vi "CurveEditor.vi"(8 "error in (no error)":errorcluster caption="entrée d'erreur (pas d'erreur)", 9 "Experiment.lvclass":refnum<class "Experiment.lvclass">=refnum, 11 "Interface en entrée":refnum<class "Interface.lvclass"> caption="Interface Class in") -> (0 "error out":errorcluster caption="sortie d'erreur", 1 "Experiment.lvclass Out":refnum<class "Experiment.lvclass">, 3 "Interface en sortie":refnum<class "Interface.lvclass"> caption="Interface Class out")   [LabVIEW 2019, in "Interface.lvclass"]
uses:
  Interface.lvclass
  Experiment Class/Experiment.lvclass
  DevicesClass/Tools/Tools.lvclass
  Calculations Class/DefaultDev_Func.ctl
  CurveSetup.ctl
  CrvEdStates.ctl
  Interface.lvclass/Interface.ctl
  <vilib>/Utility/error.llb/DialogType.ctl
  Calculations Class/Calculations.lvclass
panel:
  out "Current Task":i32=-1
  out "ScanInd":i32
  in  "AddDataSrc":bool
  in  "EditSource":i32(listbox) caption="Editing Source Curves"
  in  "Data Source 2":i32(listbox) caption="Added Operations"
  out "PanelViRefOut":refnum<vi>[](array[refnum])
  out "Point Count":i32
  out "Curve Preview":cluster{dbl[], dbl[]}[](graph)
  in  "ScanDatSrc":bool[](array[boolean])
  in  "RemOper":bool
  in  "RemDataSrc":bool
  in  "EditTask":i32(listbox) caption="Editing Task"
  in  "AddAqData":bool
  in  "Acquired Data List":i32[](listbox)
  out "2D Scan":bool
  in  "2D Plot Act":bool caption="2D Plot"
  in  "Data Only":bool
  out "GraphIndex":i32
  in  "CreateOper":bool
  in  "SaveCurvePar":bool
  in  "DisplayName":string
  out "CrvParOut":T1[](array[typedef])
  out "NomDon":string[](array[string])=["RTêta;", "X&Y;"]
  out "VarParams":string[][](array[string])
  in  "ScanParam":u16(ring) caption="Scan Parameter"
  in  "Operation":T2
  in  "stop":bool
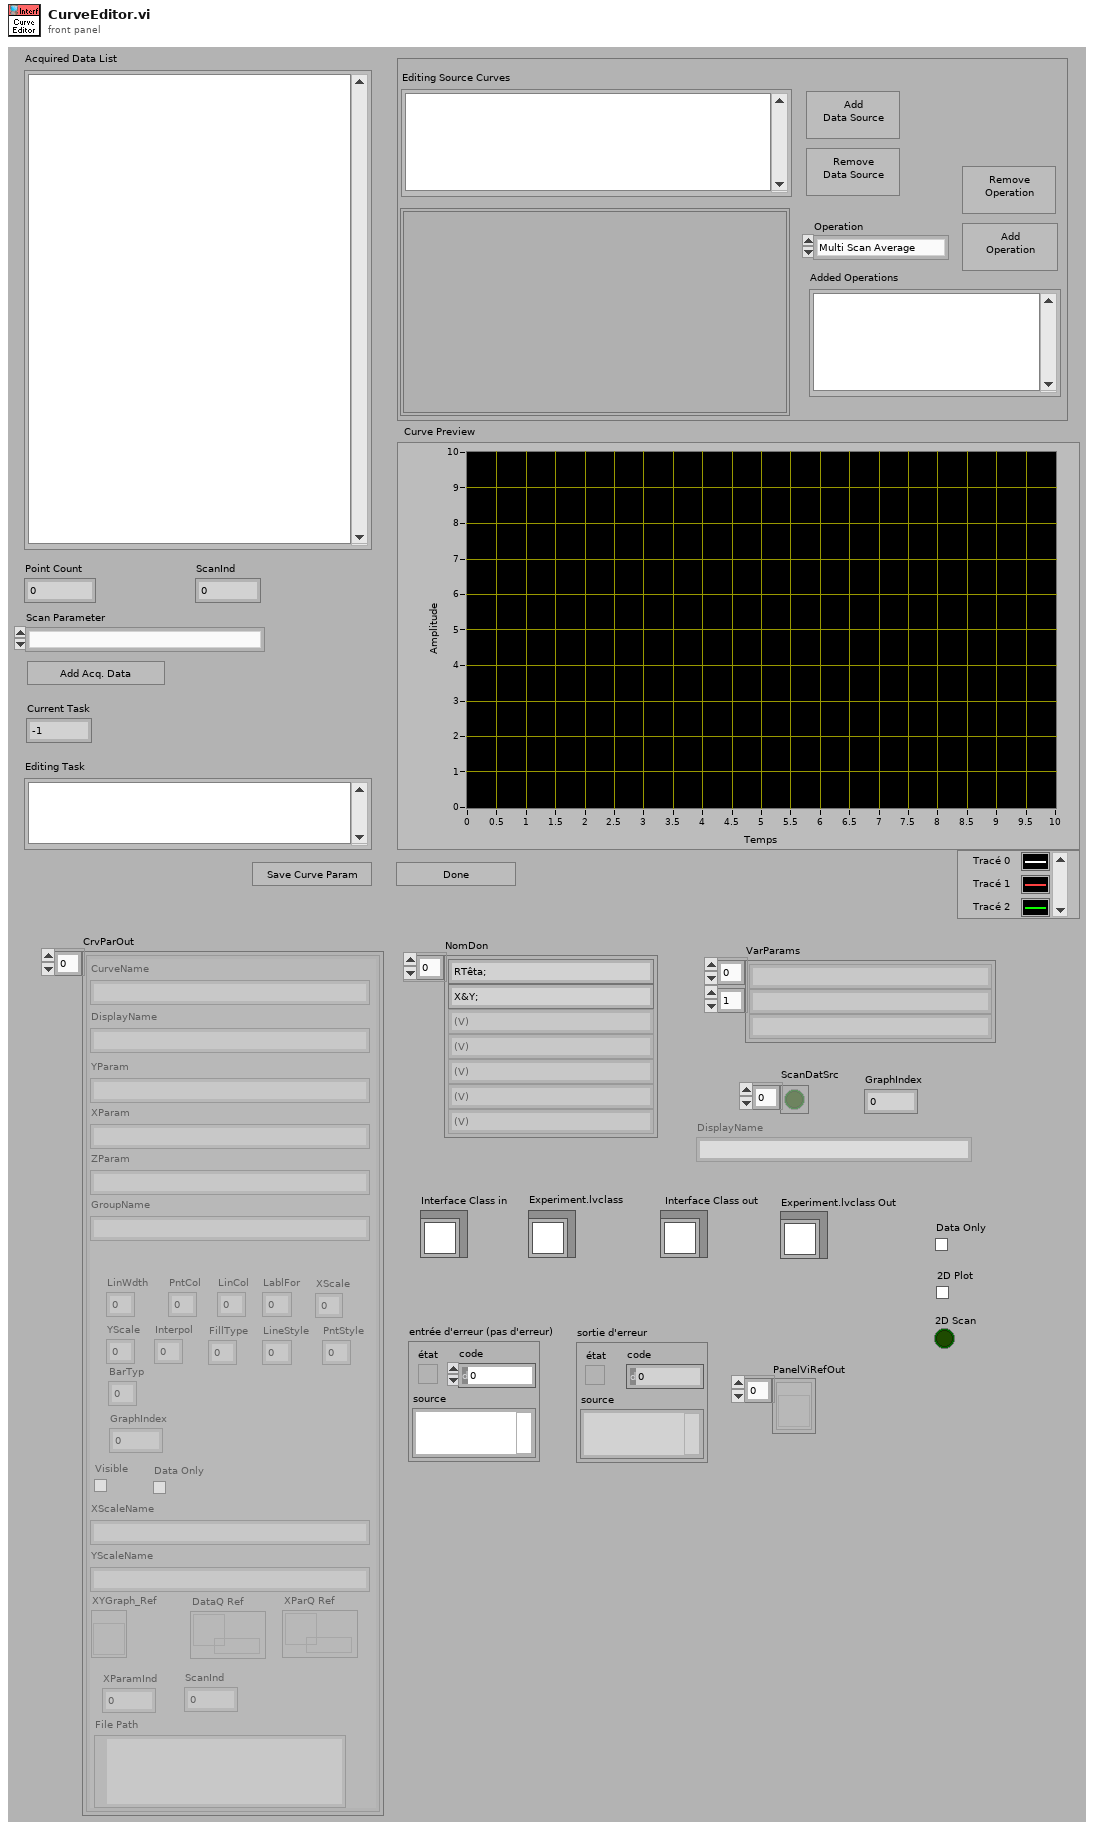
[diagram p1: front panel]
types:
  T1 = typedef "Interface.lvclass/CurveSetup.ctl" = cluster{"CurveName":string, "YParam":string, "XParam":string, "ZParam ":string, "GroupName":string, "LinWdth":u8, "PntCol":u32, "LinCol":u32, "LablFor":u8, "XScale":u32, "YScale":u32, "Interpol":u8, "DisplayName":string, "FillType":i16, "LineStyle":u8, "PntStyle":u8, "BarTyp":u8, "GraphIndex":i32, "Visible":bool, "XScaleName":string, "YScaleName":string, "XYGraph_Ref":refnum<vi>, "Data Only":bool, "DataQ Ref":refnum<queue>, "XParQ Ref":refnum<queue>, "XParamInd":i32, "ScanInd":i32, "File Path":path}
  T2 = typedef "Calculations.lvclass/DefaultDev_Func.ctl" = enum16{"Multi Scan Average", "Running Average", "Summ"}
  T3 = typedef "CrvEdStates.ctl" = enum16{"InitProg", "CreateCalc", "SaveParams", "Error", "Stop"}
  T4 = typedef "DialogType.ctl" = u16
  T5 = typedef "Interface.lvclass/ScanParams.ctl" = cluster{"Entête":string, "Scan list":string[], "NbCourbe":i32, "IndCourbe":i64, "NomDon":string[], "Session ":i32, "Date":string, "Time":string, "VarParams":string[][], "UserName":string, "ScanTableSize":i32[], "VarPar list":string[], "DescKeyword":string}
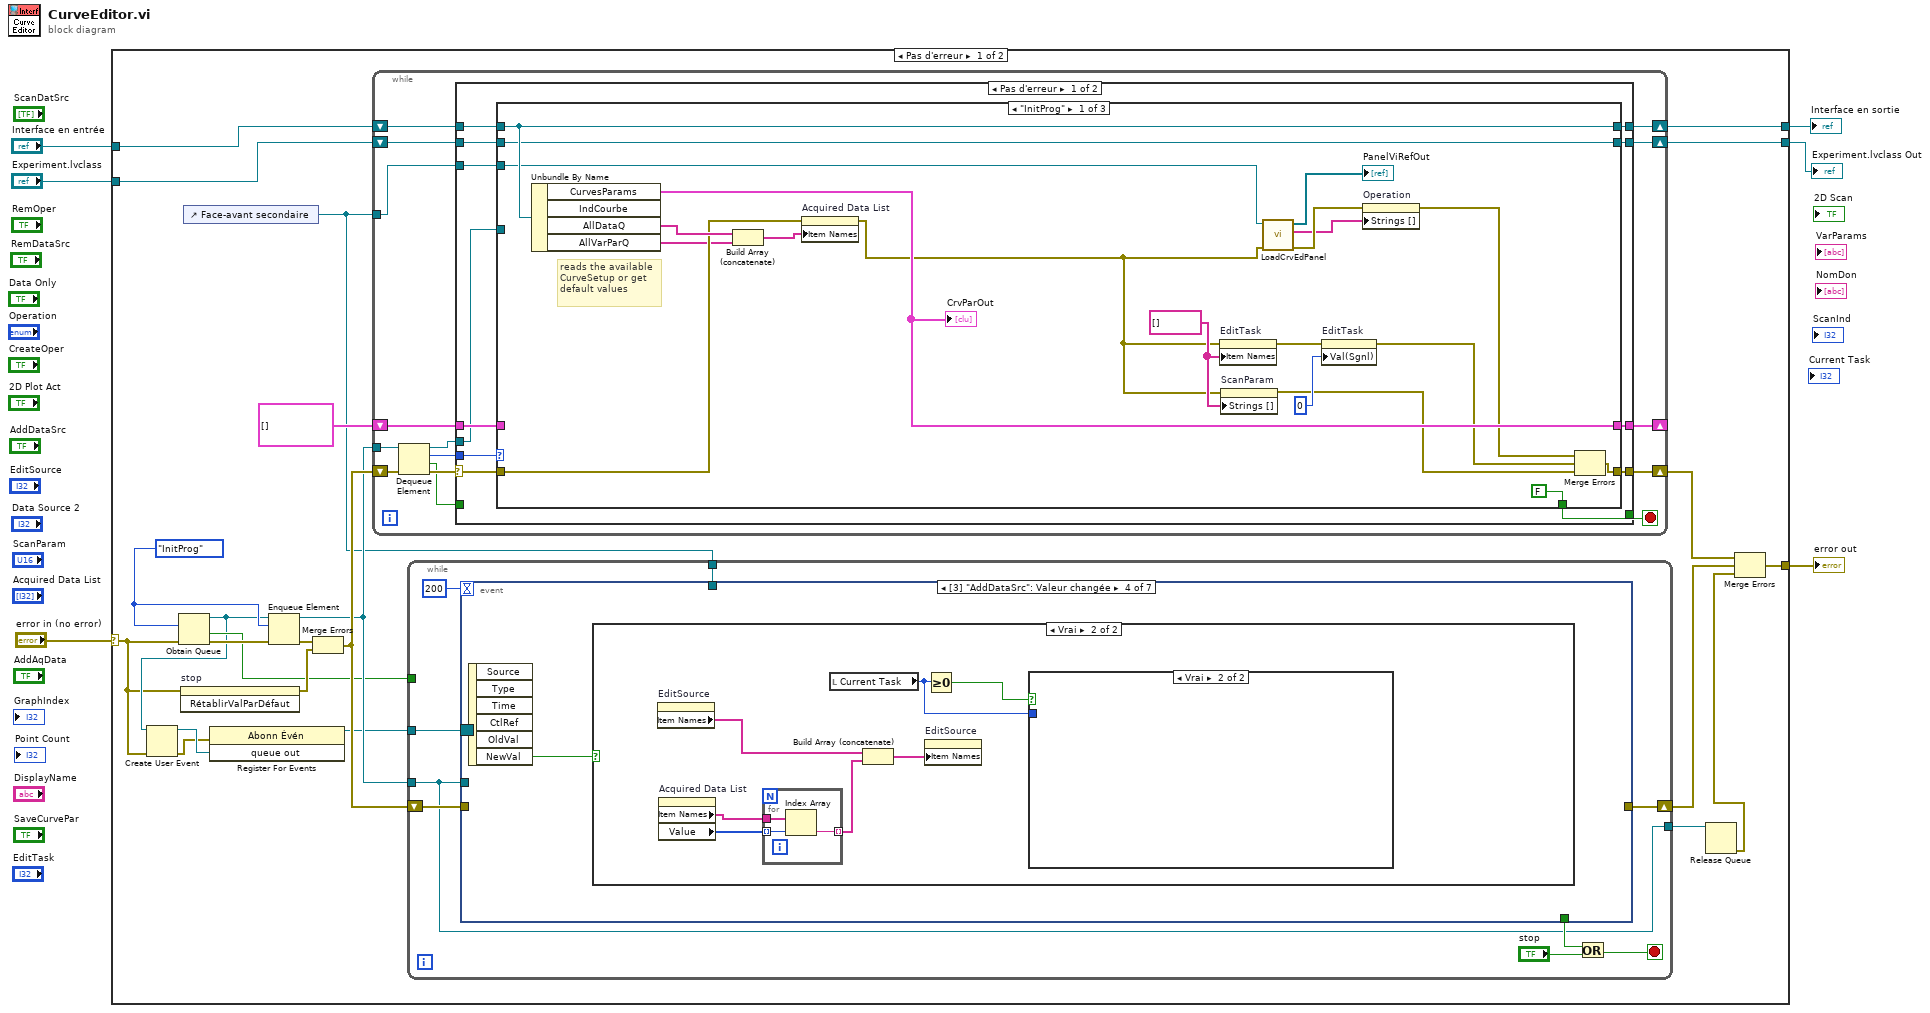
[diagram p0: block diagram]
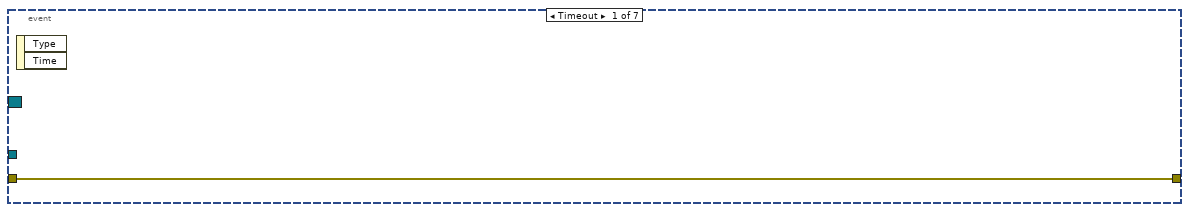
[diagram p2: hidden frame]
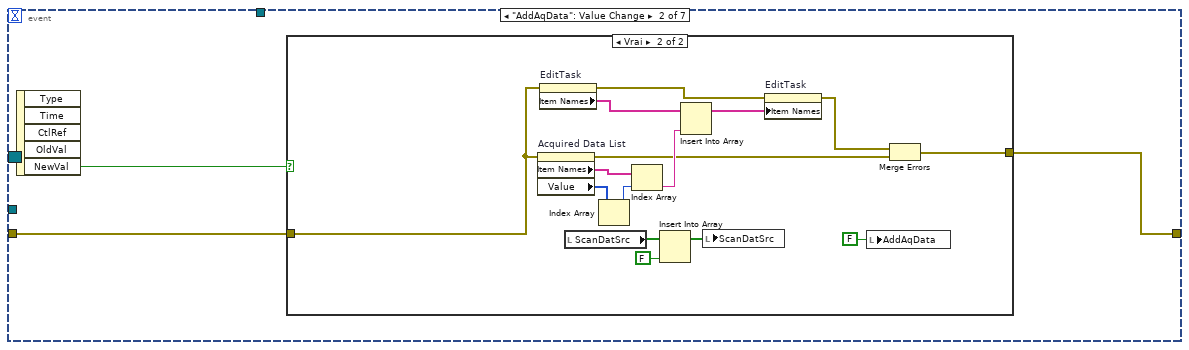
[diagram p3: hidden frame]
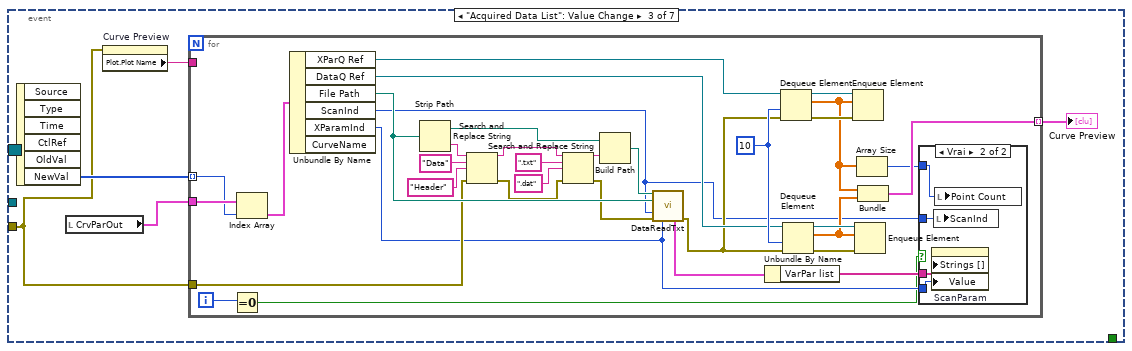
[diagram p5: hidden frame]
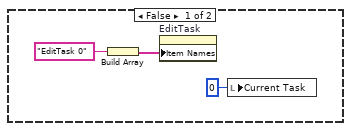
[diagram p8: hidden frame]
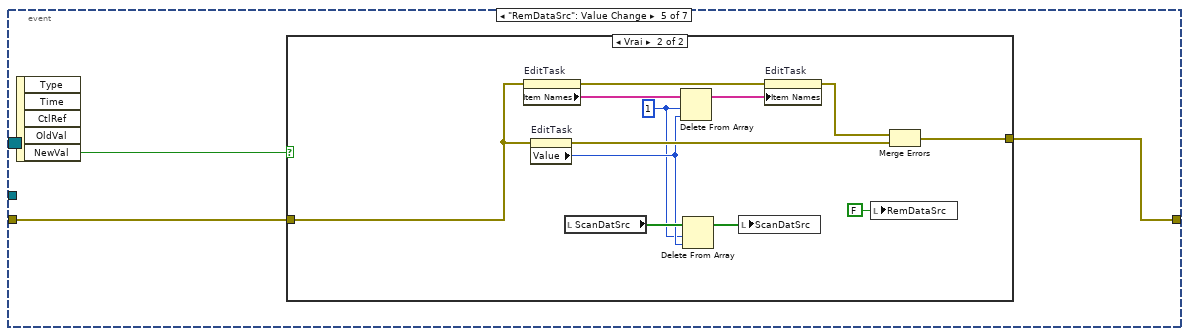
[diagram p9: hidden frame]
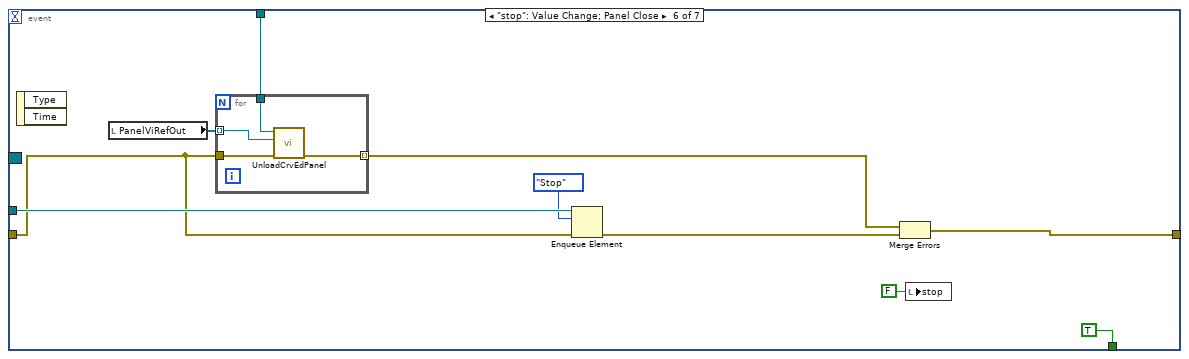
[diagram p11: hidden frame]
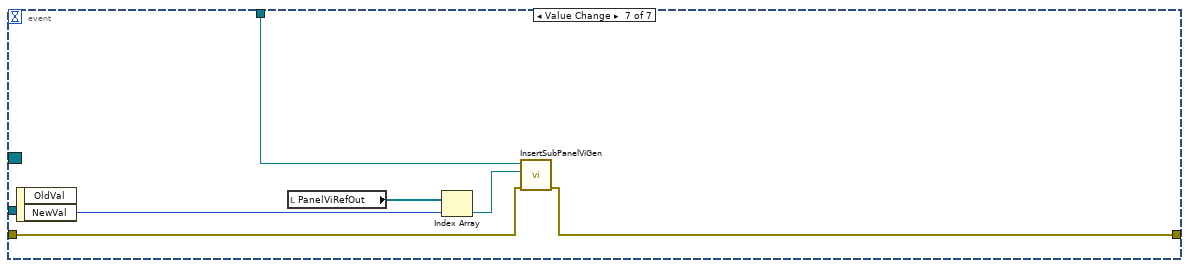
[diagram p12: hidden frame]
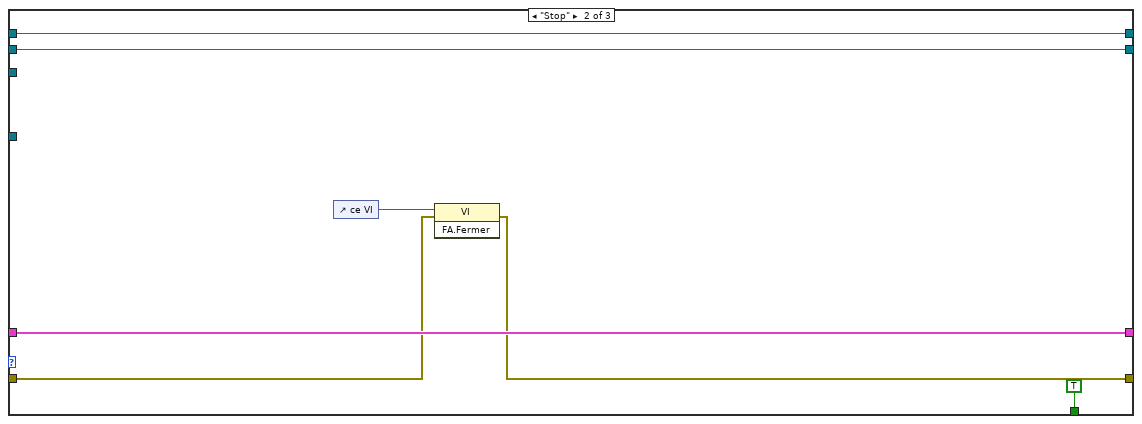
[diagram p13: hidden frame]
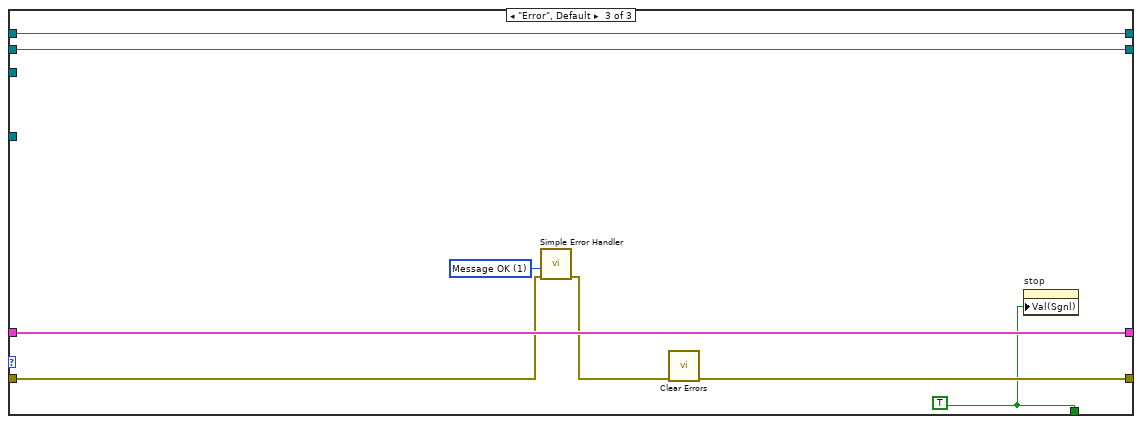
[diagram p14: hidden frame]
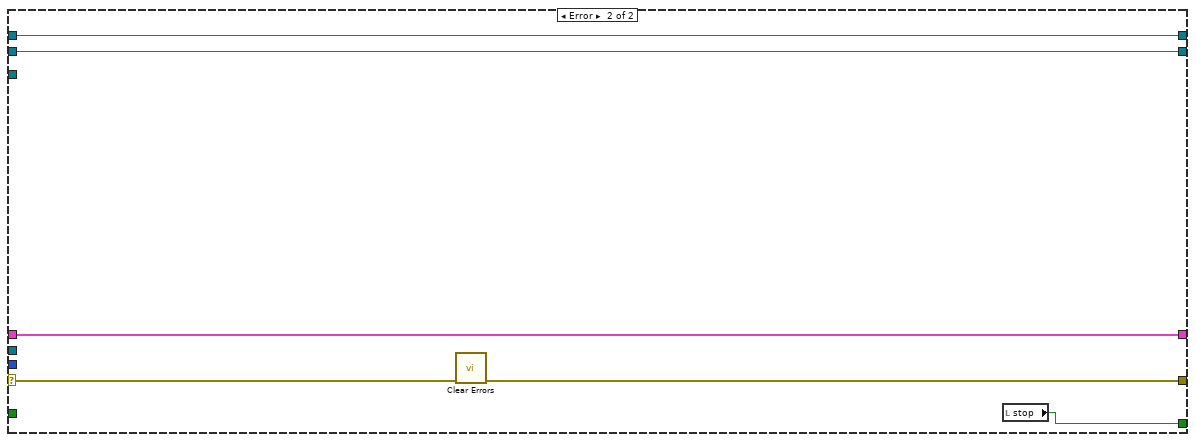
[diagram p15: hidden frame]
diagram:
  n1 = case shown="Pas d'erreur" "error in (no error)" {
    selector: "error in (no error)" -> [w11 w222]
    tunnel: [w20 w222] -> w5
    tunnel: "Interface en entrée" -> [w23 w221]
    tunnel: [w18 w221] -> w3
    tunnel: "Experiment.lvclass" -> [w28 w220]
    tunnel: [w19 w220] -> w1
    frame No Error {
      w14 = CrvEdStates."InitProg" ("Énum")
      n2 = Obtain Queue(element data type=w14, error in (no error)=w11) -> (queue out=w12:refnum<queue>, created new?=w15:bool, error out=w29:errorcluster)  [unwired: 3 in]
      n3 = Create User Event(user event datatype=w12, error in=w11) -> (user event=w10:refnum<user-event>, error out=w9:errorcluster)
      n4 = invoke on="stop" class="Bool (strict)" method="RétablirValParDéfaut"(error in=w11) -> (error out=w25:errorcluster)  [unwired: 2 in, 2 out]
      n5 = control-ref of="Face-avant secondaire"() -> (w7:refnum<vi>)
      n6 = register-events(error in=w9, w10) -> (reference out=w8:refnum<event-registration>)  [unwired: 1 in, 1 out]
      n7 = Enqueue Element(queue=w12, element=w14, error in (no error)=w29) -> (queue out=w17:refnum<queue>, error out=w26:errorcluster)  [unwired: 1 in, 1 out]
      n8 = Merge Errors(w26, w25) -> (w24:errorcluster)
      n9 = while {
        shift-right: [w160] -> w21
        shift-left: w24 -> [w166]
        tunnel: w17 -> [w157]
        shift-right: [w161] -> w18
        shift-left: w23 -> [w164]
        shift-right: [w163] -> w19
        shift-left: w28 -> [w165]
        shift-right: [w159] -> _
        shift-left: T1[] [] ("CurveParamsOut") -> [w158]
        tunnel: w7 -> [w156]
        stop <- w162 stop-if-true
        n10 = Dequeue Element(queue=w157, error in (no error)=w166) -> (queue out=w153:refnum<queue>, element=w155:T3, timed out?=w152:bool, error out=w154:errorcluster)  [unwired: 1 in]
        n11 = case shown="Pas d'erreur" w154 {
          selector: w154 -> [w168 w219]
          tunnel: w165 -> [w178 w216]
          tunnel: w164 -> [w177 w217]
          tunnel: [w176 w216] -> w163
          tunnel: [w175 w214] -> w162
          tunnel: [w174 w217] -> w161
          tunnel: [w173 w215] -> w160
          tunnel: [w172 w218] -> w159
          tunnel: w158 -> [w171 w218]
          tunnel: w156 -> [w170 _]
          tunnel: w155 -> [w169 _]
          tunnel: w153 -> [w167 _]
          tunnel: w152 -> [_ _]
          frame No Error {
            n12 = case shown="\"InitProg\"" w169 {
              tunnel: w178 -> [w191 w204 w211]
              tunnel: w177 -> [w197 w203 w212]
              tunnel: w168 -> [w189 w200 w210]
              tunnel: [w191 w204 w211] -> w176
              tunnel: [FALSE TRUE w206] -> w175
              tunnel: [w197 w203 w212] -> w174
              tunnel: [w196 w199 w208] -> w173
              tunnel: [w192 w202 w213] -> w172
              tunnel: w171 -> [_ w202 w213]
              tunnel: w167 -> [_ _ _]
              tunnel: w170 -> [w183 _ _]
              frame "InitProg" {
                w187 = string[] [] ("Item Names")
                # "reads the available CurveSetup or get default values"
                n13 = Unbundle By Name(w197) -> ("CurvesParams"=w192:T1[], "AllDataQ"=w193:string[], "AllVarParQ"=w185:string[])  [unwired: 1 out]
                "CrvParOut" <- w192
                n14 = Build Array (concatenate)(w193, w185) -> (w186:string[])
                n15 = property on="Acquired Data List" class="LstDér (strict)"(error in=w189, "Item Names"=w186) -> (error out=w184:errorcluster)  [unwired: 1 in, 1 out]
                n16 = property on="EditTask" class="LstDér (strict)"(error in=w184, "Item Names"=w187) -> (error out=w195:errorcluster)  [unwired: 1 in, 1 out]
                n17 = property on="ScanParam" class="MDér (strict)"(error in=w184, "Strings []"=w187) -> (error out=w188:errorcluster)  [unwired: 1 in, 1 out]
                n18 = call "LoadCrvEdPanel.vi"("error in (no error)"=w184, "RemPanRef"=w183) -> ("sortie d'erreur"=w182:errorcluster, "ViNameOut"=w181:string[], "PanelViRefOut"=→"PanelViRefOut":refnum<vi>[])  [unwired: 7 in]
                n19 = property on="EditTask" class="LstDér (strict)"(error in=w195, "Val(Sgnl)"=0 ("Valeur (Signalisation)")) -> (error out=w190:errorcluster)  [unwired: 1 in, 1 out]
                n20 = property on="Operation" class="Énum (strict)"(error in=w182, "Strings []"=w181) -> (error out=w180:errorcluster)  [unwired: 1 in, 1 out]
                n21 = Merge Errors(w180, w190, w188) -> (w196:errorcluster)
              }
              frame "Stop" {
                n22 = control-ref of="ce VI"() -> (w201:refnum<vi>)
                n23 = invoke class="VI" method="FA.Fermer"(reference=w201, error in=w200) -> (error out=w199:errorcluster)  [unwired: 1 in, 2 out]
              }
              frame "Error", Default {
                w206 = TRUE
                w207 = T4 1 items=["pas de dialogue", "Message OK", "Message continuer ou arrêter", "Message OK + mises en garde", "Arrêter/Continuer + mises en garde"] ("type of dialog (OK msg:1)")
                n24 = call <vilib>:"Simple Error Handler.vi"("type of dialog (OK msg:1)"=w207, "error in (no error)"=w210) -> ("error out"=w209:errorcluster)  [unwired: 3 in, 4 out]
                n25 = call <vilib>:"Clear Errors.vi"("error in (no error)"=w209) -> ("error out"=w208:errorcluster)  [unwired: 5 in, 1 out]
                n26 = property on="stop" class="Bool (strict)"("Val(Sgnl)"=w206) -> ()  [unwired: 2 in, 2 out]
              }
            }
          }
          frame Error {
            n27 = call <vilib>:"Clear Errors.vi"("error in (no error)"=w219) -> ("error out"=w215:errorcluster)  [unwired: 5 in, 1 out]
            n28 = local read "stop"() -> (w214:bool)
          }
        }
      }
      n29 = while {
        shift-right: [w36] -> w22
        shift-left: w24 -> [w37]
        tunnel: w17 -> [w32]
        tunnel: w15 -> [_]
        tunnel: [w32] -> w13
        tunnel: w8 -> [w31]
        tunnel: w7 -> [w30]
        stop <- w34 stop-if-true
        n30 = event shown="[3] \"AddDataSrc\": Valeur changée" {
          selector: w31 -> [_ _ _ _ _ _ _]
          dyn-events: _ -> [_ _ _ _ _ _ _]
          timeout: 200 -> [_ _ _ _ _ _ _]
          tunnel: w32 -> [_ _ _ _ _ w140 _]
          tunnel: w37 -> [w39 w41 w60 _ w117 w135 w150]
          tunnel: [w39 w40 _ _ w116 w136 w149] -> w36
          tunnel: [_ _ _ _ _ TRUE _] -> w33
          tunnel: w30 -> [_ _ _ _ _ w132 w151]
          event Timeout {
            n31 = event-data() -> ()  [unwired: 1 in, 2 out]
          }
          event "AddAqData": Value Change {
            n32 = event-data() -> ("NewVal"=w42:bool)  [unwired: 1 in, 4 out]
            n33 = case shown="Vrai" w42 {
              tunnel: w41 -> [w43 w51]
              tunnel: [w43 w50] -> w40
              frame False {
              }
              frame True {
                n34 = property on="Acquired Data List" class="LstDér (strict)"(error in=w51) -> (error out=w52:errorcluster, "Item Names"=w58:string[], "Value"=w45:i32[])  [unwired: 1 in, 1 out]
                n35 = property on="EditTask" class="LstDér (strict)"(error in=w51) -> (error out=w54:errorcluster, "Item Names"=w56:string[])  [unwired: 1 in, 1 out]
                n36 = local read "ScanDatSrc"() -> (w48:bool[])
                n37 = Index Array(array=w45) -> (element=w44:i32)  [unwired: 1 in]
                n38 = Index Array(array=w58, index=w44) -> (element=w57:string)
                n39 = Insert Into Array(array=w48, new element=FALSE ("new element/subarray")) -> (w47:bool[])  [unwired: 1 in]
                n40 = Insert Into Array(array=w56, new element=w57) -> (w55:string[])  [unwired: 1 in]
                n41 = local write "ScanDatSrc"(w47) -> ()
                n42 = property on="EditTask" class="LstDér (strict)"(error in=w54, "Item Names"=w55) -> (error out=w53:errorcluster)  [unwired: 1 in, 1 out]
                n43 = local write "AddAqData"(FALSE ("AddAqData")) -> ()
                n44 = Merge Errors(w53, w52) -> (w50:errorcluster)
              }
            }
          }
          event "Acquired Data List": Value Change {
            n45 = event-data() -> ("NewVal"=w61:i32[])  [unwired: 1 in, 5 out]
            n46 = local read "CrvParOut"() -> (w63:T1[])
            n47 = property on="Curve Preview" class="GraphXY (strict)"(error in=w60) -> ("Plot.Plot Name"=w59:string)  [unwired: 1 in, 2 out]
            n48 = for {
              tunnel: w63 -> [w97]
              tunnel: [w87] -> w62 mode=indexing
              tunnel: w60 -> [w78]
              tunnel: w61 -> [w66] mode=indexing
              tunnel: w59 -> [_]
              i -> [w65]
              w92 = 10 ("timeout en ms (-1)")
              n49 = Equal To 0?(x=w65) -> (x = 0?=w64:bool)
              n50 = Index Array(array=w97, index=w66) -> (element=w96:T1)
              n51 = Unbundle By Name(w96) -> ("XParQ Ref"=w89:refnum<queue>, "DataQ Ref"=w88:refnum<queue>, "File Path"=w85:path, "ScanInd"=w67:i32, "XParamInd"=w70:i32)  [unwired: 1 out]
              n52 = Strip Path(path=w85) -> (stripped path=w81:path, name=w84:string)
              n53 = Search and Replace String(input string=w84, search string="Data" ("chaîne recherchée"), replace string="Header" ("chaîne de remplacement (\"\")"), error in=w78) -> (result string=w75:string, error out=w77:errorcluster)  [unwired: 4 in, 2 out]
              n54 = Search and Replace String(input string=w75, search string=".txt" ("chaîne recherchée"), replace string=".dat" ("chaîne de remplacement (\"\")"), error in=w77) -> (result string=w73:string, error out=w74:errorcluster)  [unwired: 4 in, 2 out]
              n55 = Build Path(base path=w81, name or relative path=w73) -> (appended path=w80:path)
              n56 = call "DataReadTxt.vi"("Chemin Header"=w80, "chemin Data"=w85, "ScanlistIndex"=w67, "error in"=w74, "VarParIndex"=w70) -> ("enregistrement(s)"=w72:T5, "error out"=w86:errorcluster)  [unwired: 3 in, 6 out]
              n57 = Unbundle By Name(w72) -> ("VarPar list"=w71:string[])
              n58 = Dequeue Element(queue=w89, timeout in ms (-1)=w92, error in (no error)=w86) -> (queue out=w95:refnum<queue>, element=w69:dbl[], error out=w91:errorcluster)  [unwired: 1 out]
              n59 = Dequeue Element(queue=w88, timeout in ms (-1)=w92, error in (no error)=w86) -> (queue out=w93:refnum<queue>, element=w90:dbl[], error out=w94:errorcluster)  [unwired: 1 out]
              n60 = Enqueue Element(queue=w95, element=w69, error in (no error)=w91) -> ()  [unwired: 1 in, 3 out]
              n61 = Enqueue Element(queue=w93, element=w90, error in (no error)=w94) -> ()  [unwired: 1 in, 3 out]
              n62 = Array Size(array=w69) -> (size(s)=w68:i32)
              n63 = Bundle(w69, w90) -> (w87:cluster{dbl[], dbl[]})  [unwired: 1 in]
              n64 = case shown="Vrai" w64 {
                tunnel: w71 -> [_ w101]
                tunnel: w70 -> [_ w100]
                tunnel: w68 -> [_ w99]
                tunnel: w67 -> [_ w98]
                frame False {
                }
                frame True {
                  n65 = property on="ScanParam" class="MDér (strict)"("Strings []"=w101, "Value"=w100) -> ()  [unwired: 2 in, 2 out]
                  n66 = local write "ScanInd"(w98) -> ()
                  n67 = local write "Point Count"(w99) -> ()
                }
              }
            }
            "Curve Preview" <- w62
          }
          event "AddDataSrc": Value Change {
            n68 = event-data() -> ("NewVal"=w102:bool)  [unwired: 1 in, 5 out]
            n69 = case shown="Vrai" w102 {
              frame False {
              }
              frame True {
                n70 = property on="EditSource" class="LstDér (strict)"() -> ("Item Names"=w109:string[])  [unwired: 2 in, 2 out]
                n71 = property on="Acquired Data List" class="LstDér (strict)"() -> ("Item Names"=w107:string[], "Value"=w106:i32[])  [unwired: 2 in, 2 out]
                n72 = for {
                  tunnel: w107 -> [w115]
                  tunnel: w106 -> [w114] mode=indexing
                  tunnel: [w113] -> w105 mode=indexing
                  n73 = Index Array(array=w115, index=w114) -> (element=w113:string)
                }
                n74 = local read "Current Task"() -> (w103:i32)
                n75 = Build Array (concatenate)(w109, w105) -> (w108:string[])
                n76 = property on="EditSource" class="LstDér (strict)"("Item Names"=w108) -> ()  [unwired: 2 in, 2 out]
                n77 = Greater Or Equal To 0?(x=w103) -> (x >= 0?=w104:bool)
                n78 = case shown="Vrai" w104 {
                  tunnel: w103 -> [_ _]
                  frame False {
                    n79 = Build Array("EditTask 0") -> (w111:string[])
                    n80 = property on="EditTask" class="LstDér (strict)"("Item Names"=w111) -> ()  [unwired: 2 in, 2 out]
                    n81 = local write "Current Task"(0 ("Current Task")) -> ()
                  }
                  frame True {
                  }
                }
              }
            }
          }
          event "RemDataSrc": Value Change {
            n82 = event-data() -> ("NewVal"=w118:bool)  [unwired: 1 in, 4 out]
            n83 = case shown="Vrai" w118 {
              tunnel: w117 -> [w119 w126]
              tunnel: [w119 w125] -> w116
              frame False {
              }
              frame True {
                w120 = 1 ("length")
                n84 = property on="EditTask" class="LstDér (strict)"(error in=w126) -> (error out=w129:errorcluster, "Item Names"=w131:string[])  [unwired: 1 in, 1 out]
                n85 = property on="EditTask" class="LstDér (strict)"(error in=w126) -> (error out=w127:errorcluster, "Value"=w121:i32)  [unwired: 1 in, 1 out]
                n86 = local read "ScanDatSrc"() -> (w123:bool[])
                n87 = Delete From Array(array=w131, length=w120, index=w121) -> (array with subset deleted=w130:string[])  [unwired: 1 out]
                n88 = Delete From Array(array=w123, length=w120, index=w121) -> (array with subset deleted=w122:bool[])  [unwired: 1 out]
                n89 = local write "ScanDatSrc"(w122) -> ()
                n90 = property on="EditTask" class="LstDér (strict)"(error in=w129, "Item Names"=w130) -> (error out=w128:errorcluster)  [unwired: 1 in, 1 out]
                n91 = local write "RemDataSrc"(FALSE ("AddDataSrc")) -> ()
                n92 = Merge Errors(w128, w127) -> (w125:errorcluster)
              }
            }
          }
          event "stop": Value Change; Panel Close {
            n93 = event-data() -> ()  [unwired: 1 in, 2 out]
            n94 = local read "PanelViRefOut"() -> (w133:refnum<vi>[])
            n95 = for {
              tunnel: w135 -> [w145]
              tunnel: [w144] -> w134 mode=indexing
              tunnel: w133 -> [w143] mode=indexing
              tunnel: w132 -> [w142]
              n96 = call "UnloadCrvEdPanel.vi"("error in (no error)"=w145, "CrvEdViRef"=w143, "RemPanRef"=w142) -> ("error out"=w144:errorcluster)  [unwired: 8 in]
            }
            n97 = Enqueue Element(queue=w140, element=CrvEdStates."Stop" ("Énum"), error in (no error)=w135) -> (error out=w141:errorcluster)  [unwired: 1 in, 2 out]
            n98 = Merge Errors(w134, w141) -> (w136:errorcluster)
            n99 = local write "stop"(FALSE ("stop")) -> ()
          }
          event Value Change {
            n100 = event-data() -> ("NewVal"=w146:T2)  [unwired: 1 in, 1 out]
            n101 = local read "PanelViRefOut"() -> (w148:refnum<vi>[])
            n102 = Index Array(array=w148, index=w146) -> (element=w147:refnum<vi>)
            n103 = call <userlib>:"InsertSubPanelViGen.vi"("error in (no error)"=w150, "RemVIRef"=w147, "RemPanRef"=w151) -> ("sortie d'erreur"=w149:errorcluster)  [unwired: 6 in, 2 out]
          }
        }
        n104 = Or(x=w33, y="stop") -> (x .or. y?=w34:bool)
      }
      n105 = Release Queue(queue=w13) -> (error out=w16:errorcluster)  [unwired: 2 in, 2 out]
      n106 = Merge Errors(w21, w22, w16) -> (w20:errorcluster)
    }
    frame Error {
    }
  }
  "error out" <- w5
  "Interface en sortie" <- w3
  "Experiment.lvclass Out" <- w1
